vi "CRYMulti Excel Export.vi"(5 "Excel path":path, 6 "Datafile path":path, 7 "New/Append":string, 8 "Comment":string, 9 "Format info":T1, 10 "Curves list to save":string[](array[string]), 11 "Is results? (T)":bool) -> (0 "error out":errorcluster)   [LabVIEW 2013]
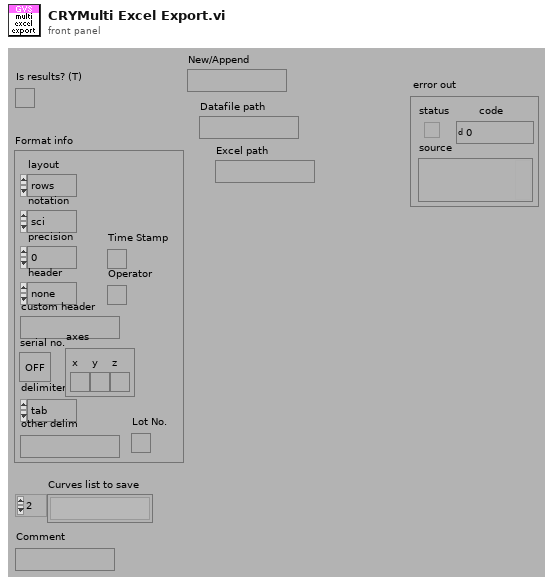
[diagram p1: front panel]
types:
  T1 = cluster{"layout":enum16{"rows", "columns"}, "notation":enum16{"sci", "float"}, "precision":i32, "header":enum16{"none", "standard", "custom"}, "custom header":string, "serial no.":bool, "delimiter":enum16{"tab", "comma", "space", "other"}, "other delim":string, "axes":cluster{"x":bool, "y":bool, "z":bool}, "Lot No.":bool, "Operator":bool, "Time Stamp":bool}
  T2 = typedef "CRYData Cluster.ctl" = cluster{"Name":string, "Curve":cluster{"x":dbl, "y":dbl, "z":dbl}[], "X data":u16, "Y data":u16, "Z data":u16, "X axis":u16, "Y axis":u16, "Z axis":u16, "X unit":string, "Y unit":string, "Z unit":string, "X dB ref":dbl, "Y dB ref":dbl, "Z dB ref":dbl, "single val":bool, "protected":bool, "display X":bool, "display Y":bool, "display Z":bool, "Test Info":string, "Step No.":i32, "Plot Settings":cluster{"Color":u32, "Interpolation":u8, "Point Style":u8, "Line Style":u8, "Point Color":u32, "Line Width":u8, "Bar Plot Style":u8, "Fill To":i16}, "AutoProtect":bool}
  T3 = typedef "CRYResult Cluster.ctl" = cluster{"Name":string, "Margin":dbl, "unit":string, "Verdict":bool, "Limit":string, "Max/Min":string, "protected":bool, "Step No.":i32, "Test Info":string, "AutoProtect":bool}
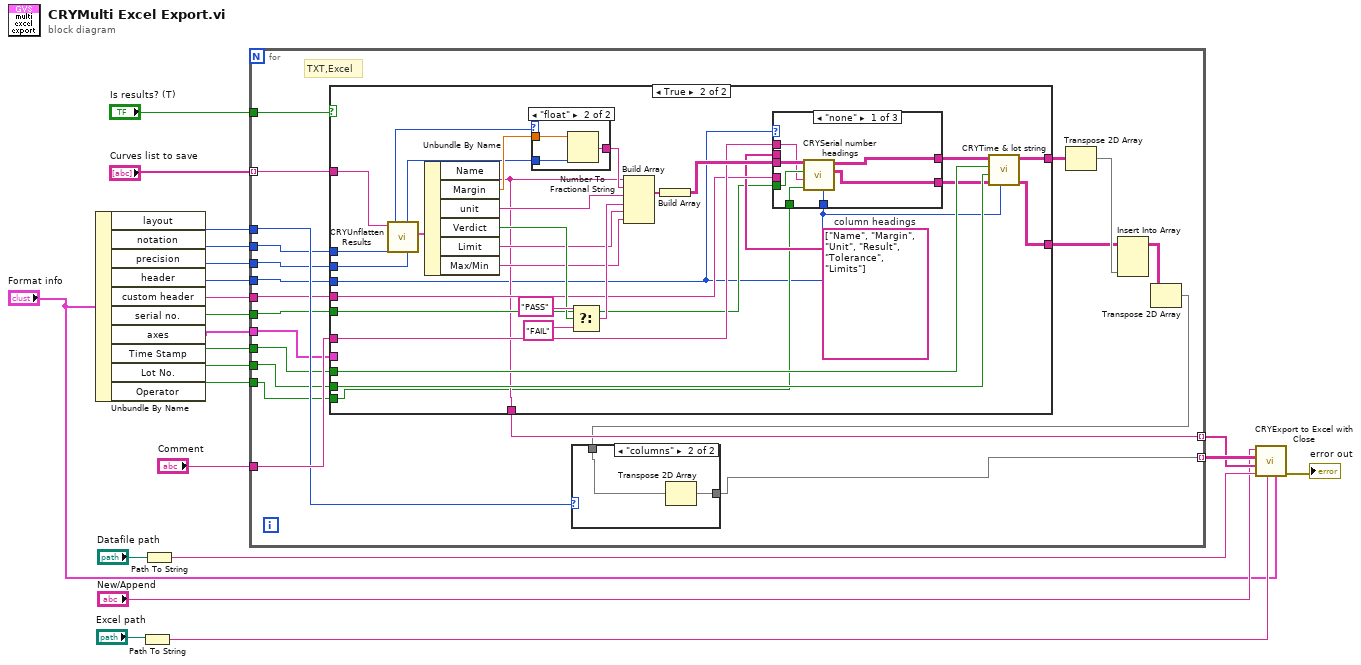
[diagram p0: block diagram]
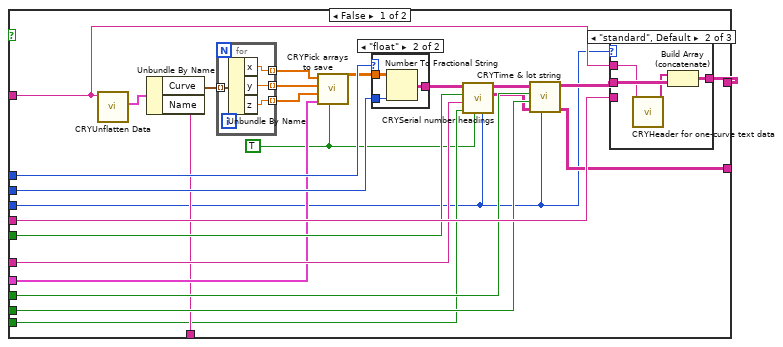
[diagram p3: hidden frame]
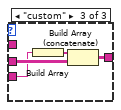
[diagram p5: hidden frame]
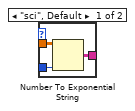
[diagram p6: hidden frame]
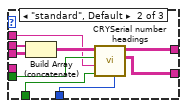
[diagram p7: hidden frame]
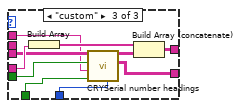
[diagram p8: hidden frame]
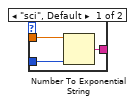
[diagram p9: hidden frame]
diagram:
  n1 = Unbundle By Name("Format info") -> ("layout"=w1:enum16{"rows", "columns"}, "notation"=w12:enum16{"sci", "float"}, "precision"=w11:i32, "header"=w10:enum16{"none", "standard", "custom"}, "custom header"=w9:string, "serial no."=w8:bool, "axes"=w7:cluster{"x":bool, "y":bool, "z":bool}, "Time Stamp"=w6:bool, "Lot No."=w5:bool, "Operator"=w3:bool)
  n2 = Path To String(path="Excel path") -> (string=w13:string)
  n3 = Path To String(path="Datafile path") -> (string=w19:string)
  n4 = for {
    tunnel: "Curves list to save" -> [w42] mode=indexing
    tunnel: "Is results? (T)" -> [w41]
    tunnel: [w40] -> w17 mode=indexing
    tunnel: [w39] -> w16 mode=indexing
    tunnel: w1 -> [w37]
    tunnel: w12 -> [w36]
    tunnel: w11 -> [w35]
    tunnel: w10 -> [w34]
    tunnel: w9 -> [w33]
    tunnel: w8 -> [w32]
    tunnel: w7 -> [w31]
    tunnel: w6 -> [w30]
    tunnel: w5 -> [w29]
    tunnel: "Comment" -> [w38]
    tunnel: w3 -> [w23]
    # "TXT,Excel"
    n5 = case shown="True" w41 {
      tunnel: w35 -> [w68 w102]
      tunnel: w36 -> [w67 w101]
      tunnel: w34 -> [w46 w90]
      tunnel: w33 -> [w66 w104]
      tunnel: w38 -> [w61 w105]
      tunnel: w42 -> [w65 w108]
      tunnel: [w64 w95] -> w26
      tunnel: w32 -> [w62 w100]
      tunnel: w31 -> [w57 _]
      tunnel: w30 -> [w54 w97]
      tunnel: w29 -> [w53 w96]
      tunnel: [w51 w94] -> w39
      tunnel: [w49 w92] -> w25
      tunnel: w23 -> [w48 w91]
      frame False {
        w47 = TRUE ("Start of file")
        n6 = call "CRYUnflatten Data.vi"("Unflatten data"=w65) -> ("Datum"=w69:T2)  [unwired: 8 in, 2 out]
        n7 = Unbundle By Name(w69) -> ("Curve"=w70:cluster{"x":dbl, "y":dbl, "z":dbl}[], "Name"=w51:string)
        n8 = for {
          tunnel: w70 -> [w89] mode=indexing
          tunnel: [w88] -> w60 mode=indexing
          tunnel: [w87] -> w59 mode=indexing
          tunnel: [w86] -> w58 mode=indexing
          n9 = Unbundle By Name(w89) -> ("x"=w88:dbl, "y"=w87:dbl, "z"=w86:dbl)
        }
        n10 = call "CRYPick arrays to save.vi"("Start of file"=w47, "axes"=w57, "Z"=w58, "Y"=w59, "X"=w60) -> ("Data points to save"=w56:dbl[][])  [unwired: 6 in]
        n11 = case shown="\"float\"" w67 {
          tunnel: w56 -> [w82 w85]
          tunnel: w68 -> [w81 w84]
          tunnel: [w80 w83] -> w63
          frame "sci", Default {
            n12 = Number To Exponential String(number=w82, precision (6)=w81) -> (E-format string=w80:string[][])  [unwired: 2 out]
          }
          frame "float" {
            n13 = Number To Fractional String(number=w85, precision (6)=w84) -> (F-format string=w83:string[][])  [unwired: 2 out]
          }
        }
        n14 = call "CRYSerial number headings.vi"("header"=w46, "Start of file"=w47, "Operator"=w48, "Comment"=w61, "Include serial numbers (F)"=w62, "Table in"=w63) -> ("Header out"=w50:string[][], "Table out"=w55:string[][])  [unwired: 4 in]
        n15 = call "CRYTime & lot string.vi"("header"=w46, "Header in"=w50, "Lot No."=w53, "Time Stamp"=w54, "Table in"=w55) -> ("Header out"=w49:string[][], "Table out"=w52:string[][])  [unwired: 3 in, 2 out]
        n16 = case shown="\"standard\", Default" w46 {
          tunnel: w52 -> [w71 w75 w79]
          tunnel: [w71 w74 w78] -> w64
          tunnel: w66 -> [_ _ w77]
          tunnel: w65 -> [_ w72 _]
          frame "none" {
          }
          frame "standard", Default {
            n17 = call "CRYHeader for one-curve text data.vi"("Data curve, flat"=w72) -> ("Header row"=w73:string[])  [unwired: 10 in]
            n18 = Build Array (concatenate)(w73, w75) -> (w74:string[][])
          }
          frame "custom" {
            n19 = Build Array(w77) -> (w76:string[])
            n20 = Build Array (concatenate)(w76, w79) -> (w78:string[][])
          }
        }
      }
      frame True {
        w103 = string[] ["Name", "Margin", "Unit", "Result", "Tolerance", "Limits"]  # column headings
        n21 = call "CRYUnflatten Results.vi"("Unflatten Result"=w108) -> ("Result"=w117:T3)  [unwired: 8 in, 2 out]
        n22 = Unbundle By Name(w117) -> ("Name"=w94:string, "Margin"=w111:dbl, "unit"=w99:string, "Verdict"=w114:bool, "Limit"=w112:string, "Max/Min"=w109:string)
        n23 = case shown="\"float\"" w101 {
          tunnel: w111 -> [w146 w149]
          tunnel: w102 -> [w145 w148]
          tunnel: [w144 w147] -> w110
          frame "sci", Default {
            n24 = Number To Exponential String(number=w146, precision (6)=w145) -> (E-format string=w144:string)  [unwired: 2 out]
          }
          frame "float" {
            n25 = Number To Fractional String(number=w149, precision (6)=w148) -> (F-format string=w147:string)  [unwired: 2 out]
          }
        }
        n26 = Select(t="PASS", s=w114, f="FAIL") -> (s? t:f=w113:string)
        n27 = Build Array(w94, w110, w99, w113, w112, w109) -> (w107:string[])
        n28 = Build Array(w107) -> (w106:string[][])
        n29 = case shown="\"none\"" w90 {
          tunnel: w103 -> [_ w133 _]
          tunnel: w106 -> [w124 w132 w140]
          tunnel: [w123 w130 w143] -> w98
          tunnel: w104 -> [_ _ w142]
          tunnel: w105 -> [w121 w128 w137]
          tunnel: w100 -> [w122 w129 w138]
          tunnel: [w120 w127 w136] -> w93
          tunnel: w91 -> [w119 w126 w135]
          tunnel: w90 -> [w118 w125 w134]
          frame "none" {
            n30 = call "CRYSerial number headings.vi"("header"=w118, "Operator"=w119, "Comment"=w121, "Include serial numbers (F)"=w122, "Table in"=w124) -> ("Header out"=w120:string[][], "Table out"=w123:string[][])  [unwired: 5 in]
          }
          frame "standard", Default {
            n31 = Build Array (concatenate)(w133, w132) -> (w131:string[][])
            n32 = call "CRYSerial number headings.vi"("header"=w125, "Operator"=w126, "Comment"=w128, "Include serial numbers (F)"=w129, "Table in"=w131) -> ("Header out"=w127:string[][], "Table out"=w130:string[][])  [unwired: 5 in]
          }
          frame "custom" {
            n33 = Build Array(w142) -> (w141:string[])
            n34 = call "CRYSerial number headings.vi"("header"=w134, "Operator"=w135, "Comment"=w137, "Include serial numbers (F)"=w138, "Table in"=w140) -> ("Header out"=w136:string[][], "Table out"=w139:string[][])  [unwired: 5 in]
            n35 = Build Array (concatenate)(w141, w139) -> (w143:string[][])
          }
        }
        n36 = call "CRYTime & lot string.vi"("header"=w90, "Header in"=w93, "Lot No."=w96, "Time Stamp"=w97, "Table in"=w98) -> ("Header out"=w92:string[][], "Table out"=w95:string[][])  [unwired: 3 in, 2 out]
      }
    }
    n37 = Transpose 2D Array(2D array=w26) -> (transposed array=w27:string[][])
    n38 = Insert Into Array(array=w25, new element=w27) -> (w28:string[][])  [unwired: 2 in]
    n39 = Transpose 2D Array(2D array=w28) -> (transposed array=w24:string[][])
    n40 = case shown="\"columns\"" w37 {
      tunnel: w24 -> [w43 w45]
      tunnel: [w43 w44] -> w40
      frame "rows", Default {
      }
      frame "columns" {
        n41 = Transpose 2D Array(2D array=w45) -> (transposed array=w44:string[][])
      }
    }
  }
  n42 = call "CRYExport to Excel with Close.vi"("Format info"="Format info", "ExcelPath"=w13, "FilePath"=w19, "Sheet Names"=w16, "Data"=w17, "New/Append"="New/Append") -> ("error out"=→"error out":errorcluster)  [unwired: 5 in]
